vi "Delete Instr.vi"(0 "Setup":T1[](array[typedef]) {"Private"."Offset" format="%^_3e"; "Private"."Scale Factors" format="%^_3e"}, 1 "Item Names":string[](array[string]), 2 "Instrument List":i32) -> (3 "Setup Out":T1[](array[typedef]) {"Private"."Offset" format="%^_3e"; "Private"."Scale Factors" format="%^_3e"}, 4 "Item Names Out":string[](array[string]), 6 "Instrument List Out":i32)   [LabVIEW 2021]
uses:
  New NML Data Acq/Sub Controls/Instrument Properties.ctl
  New NML Data Acq/Sub Controls/Public.ctl
  New NML Data Acq/Sub Controls/Private.ctl
  New NML Data Acq/Sub Controls/Instrument Ref.ctl
  New NML Data Acq/Sub Controls/SystemCheckBox-resize.ctl
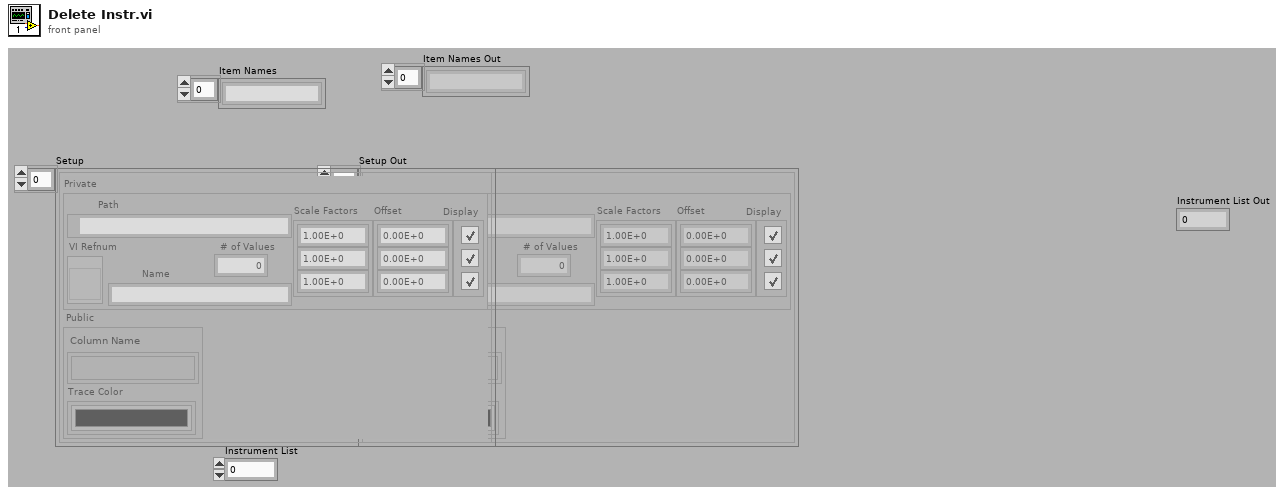
[diagram p1: front panel]
types:
  T1 = typedef "Instrument Properties.ctl" = cluster{"Public":T2, "Private":T3}
  T2 = typedef "Public.ctl" = cluster{"Column Name":string[], "Trace Color":u32[]}
  T3 = typedef "Private.ctl" = cluster{"Path":path, "VI Refnum":T4, "Name":string, "# of Values":i32, "Scale Factors":dbl[], "Display":T5[], "Offset":dbl[]}
  T4 = typedef "Instrument Ref.ctl" = refnum<vi>
  T5 = typedef "SystemCheckBox-resize.ctl" = bool
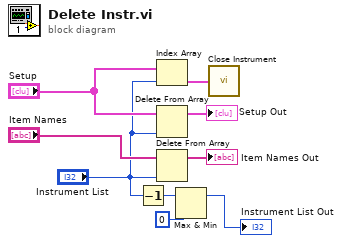
[diagram p0: block diagram]
diagram:
  n1 = Decrement(x="Instrument List") -> (x-1=w6:i32)
  n2 = Index Array(array="Setup", index="Instrument List") -> (element=w1:T1)
  n3 = Delete From Array(array="Setup", index="Instrument List") -> (array with subset deleted=→"Setup Out":T1[])  [unwired: 1 in, 1 out]
  n4 = Delete From Array(array="Item Names", index="Instrument List") -> (array with subset deleted=→"Item Names Out":string[])  [unwired: 1 in, 1 out]
  n5 = Max & Min(x=w6, y=0) -> (max(x,y)=→"Instrument List Out":i32)  [unwired: 1 out]
  n6 = call "Close Instrument.vi"("Instrument Prop"=w1) -> ()  [unwired: 1 out]
